vi "Tosca-Short Histogram Names.vi"(7 "Names":string[](array[string])) -> (8 "Short names":string[](array[string]))   [LabVIEW 2020]
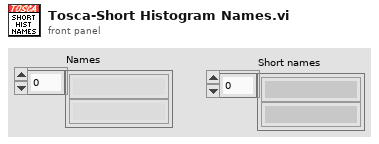
[diagram p1: front panel]
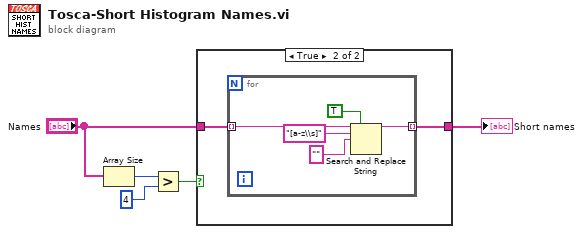
[diagram p0: block diagram]
diagram:
  n1 = Array Size(array="Names") -> (size(s)=w5:i32)
  n2 = Greater?(x=w5, y=4) -> (0:w2:bool)
  n3 = case shown="True" w2 {
    tunnel: "Names" -> [w6 w8]
    tunnel: [w6 w7] -> w1
    frame False {
    }
    frame True {
      n4 = for {
        tunnel: w8 -> [w13] mode=indexing
        tunnel: [w12] -> w7 mode=indexing
        n5 = Search and Replace String(replace all?=TRUE ("replace all? (F)"), input string=w13, search string="[a-z\\s]", replace string="" ("replace string (\"\")")) -> (result string=w12:string)  [unwired: 4 in, 3 out]
      }
    }
  }
  "Short names" <- w1
